vi "Logging Message Loop.vi"(8 "error in (no error)":errorcluster, 10 "Data Queue":refnum<queue>, 11 "Message Queues":T1) -> (0 "error out":errorcluster)   [LabVIEW 2019, in "Logging.lvlib"]
doc: "The message loop subVI to handle messages pertaining to logging data."
uses:
  Logging.lvlib
  support/Message Queue/All Message Queues.ctl
  support/Message Queue/Message Cluster.ctl
  controls/Components Message Queues.ctl
  Logging Configuration.ctl
  Logging State.ctl
  support/Message Queue/Enqueue Message (Single).vi
  <vilib>/Utility/error.llb/Error Cluster From Error Code.vi
  <vilib>/ErrorRing/Error Ring.xnode
  support/Message Queue/Message Queue.lvlib
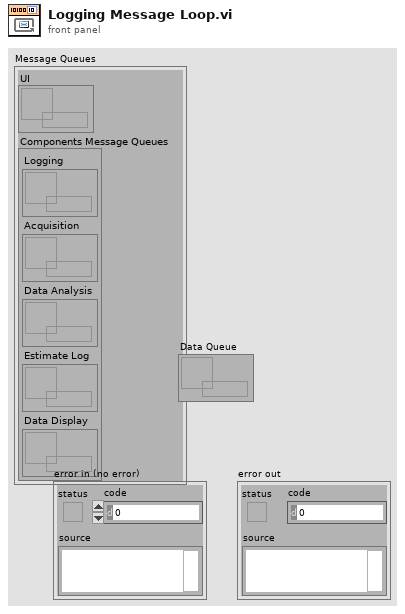
[diagram p1: front panel]
types:
  T1 = typedef "Message Queue.lvlib/All Message Queues.ctl" = cluster{"UI":refnum<queue>, "Components Message Queues":T2}
  T2 = typedef "Message Queue.lvlib/Components Message Queues.ctl" = cluster{"Logging":refnum<queue>, "Acquisition":refnum<queue>, "Data Analysis":refnum<queue>, "Estimate Log":refnum<queue>, "Data Display":refnum<queue>}
  T3 = typedef "Logging.lvlib/Logging State.ctl" = cluster{"State":enum16{"Logging", "Not Logging", "Idle"}, "Samples to Save":u32, "Force Trigger":bool}
  T4 = typedef "Logging.lvlib/Logging Configuration.ctl" = cluster{"Log File Base Path":path, "DAQ Log TDMS File Reference":refnum<k34>, "Samples to Save":u32, "Trigger - Time":u32, "Trigger - Threshold":dbl, "Trigger - Channel":u32, "Enable Time Trigger":bool, "Enable Threshold Trigger":bool, "Always Log":bool, "Session Name":string}
  T5 = enum16{"open", "open or create", "create or replace", "create", "open (read-only)"}
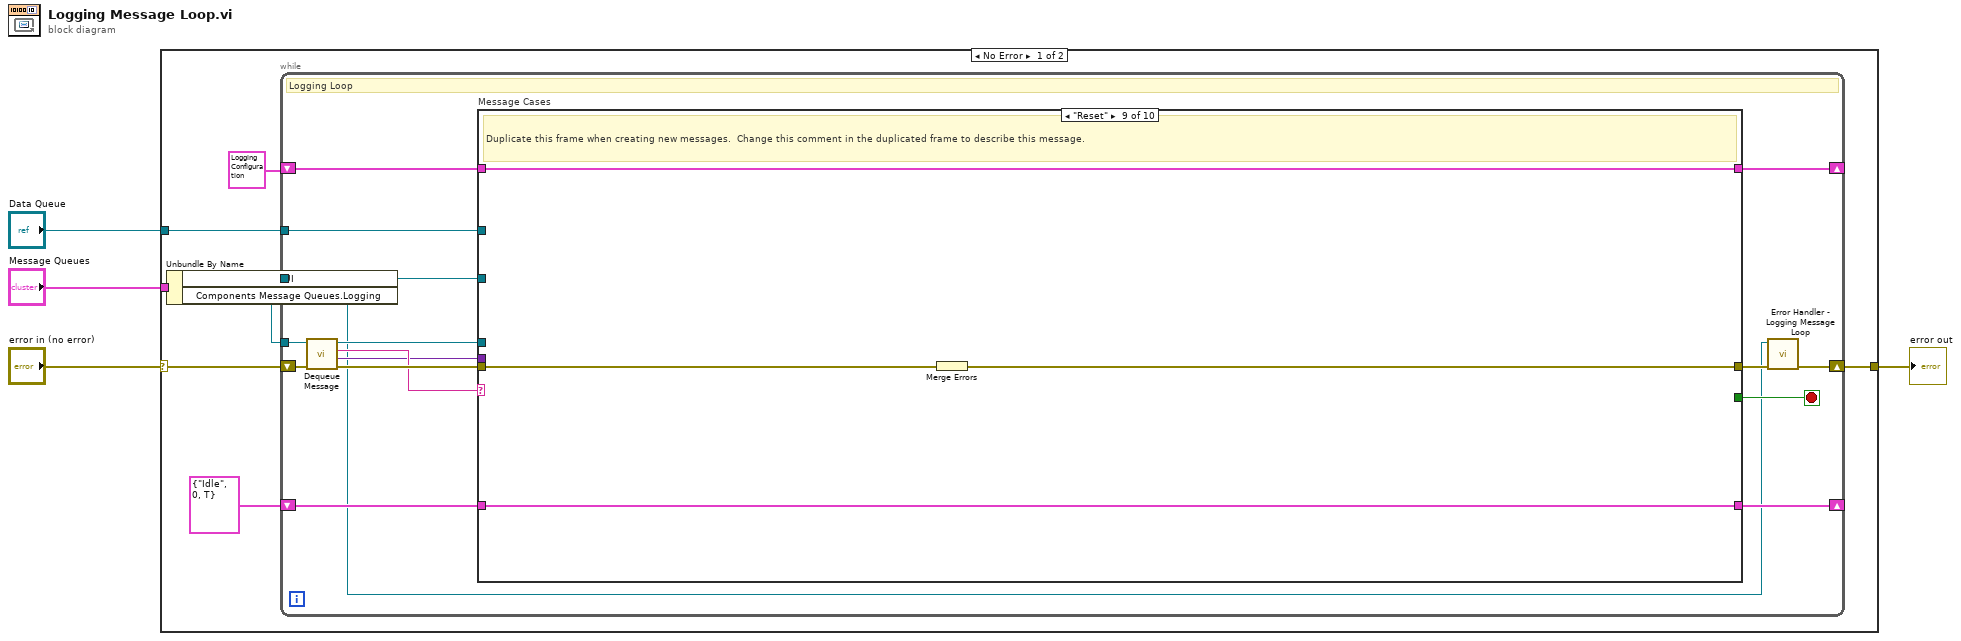
[diagram p0: block diagram]
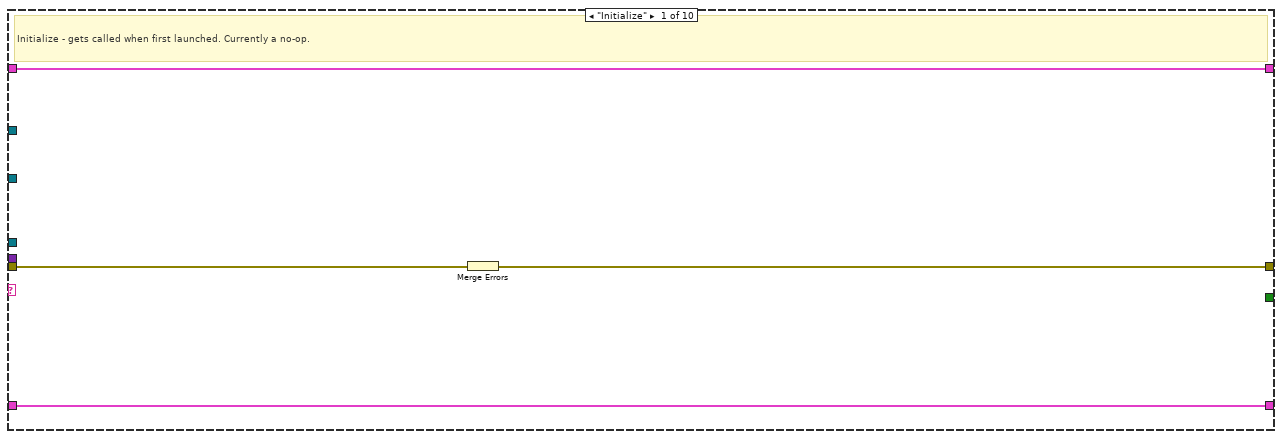
[diagram p2: hidden frame]
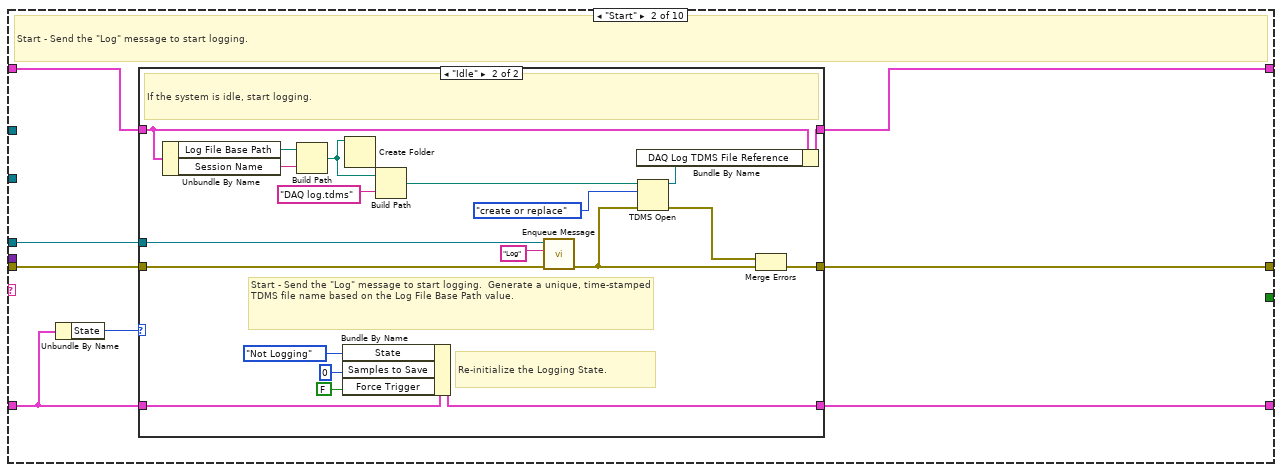
[diagram p3: hidden frame]
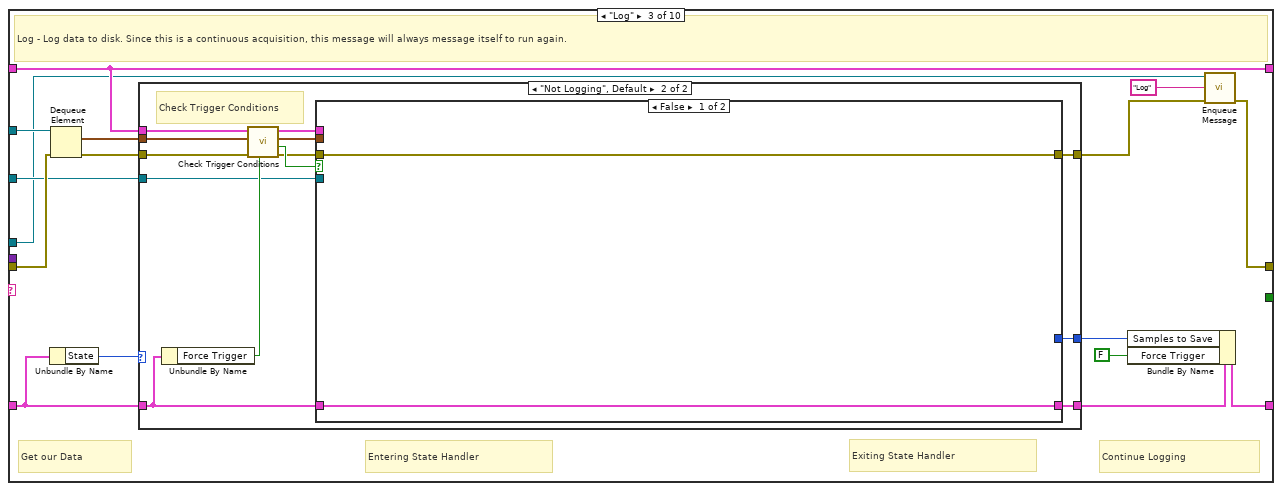
[diagram p5: hidden frame]
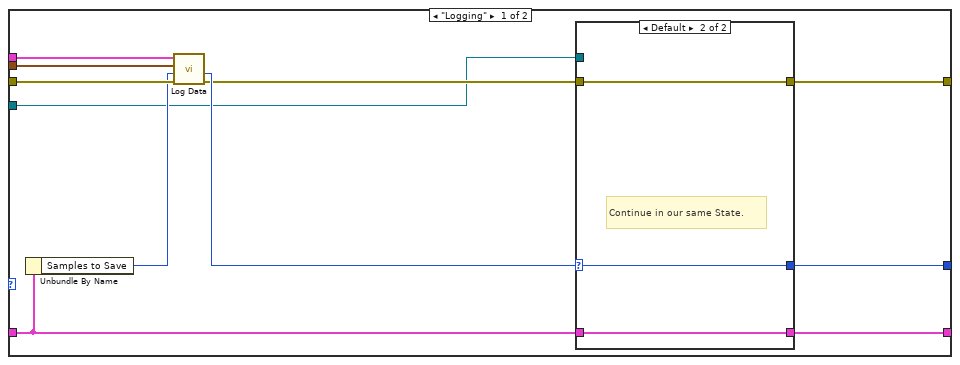
[diagram p6: hidden frame]
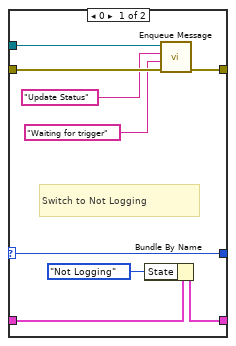
[diagram p7: hidden frame]
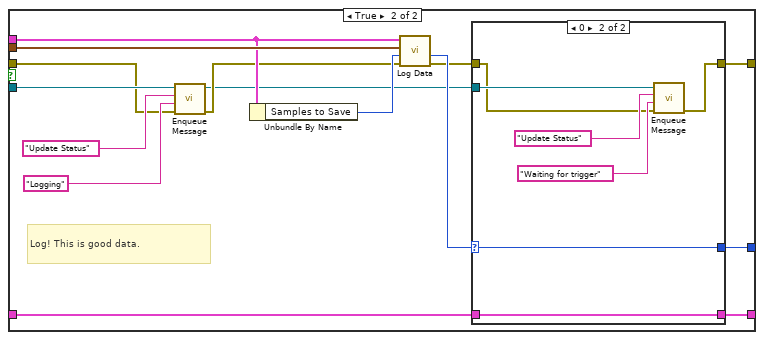
[diagram p8: hidden frame]
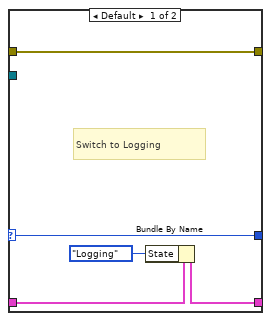
[diagram p9: hidden frame]
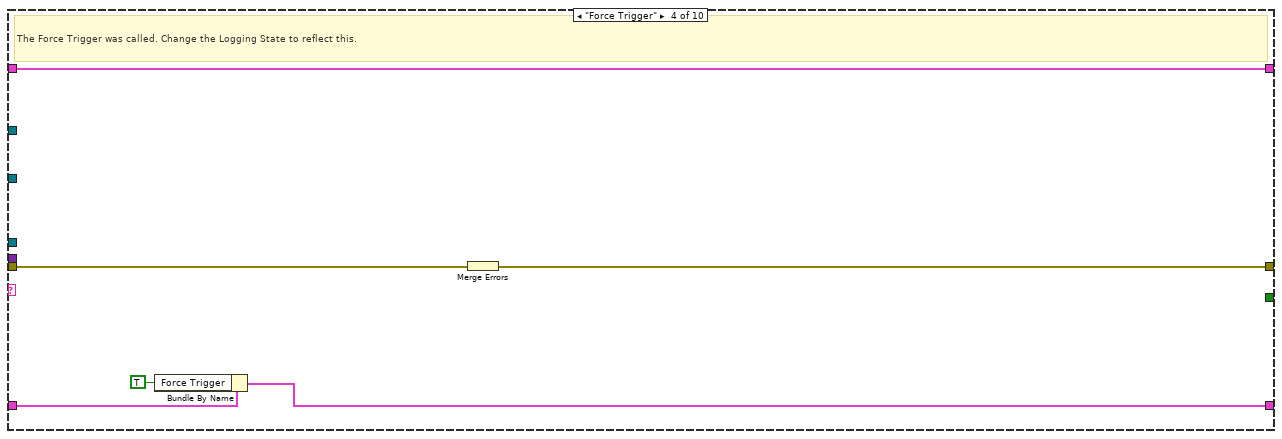
[diagram p10: hidden frame]
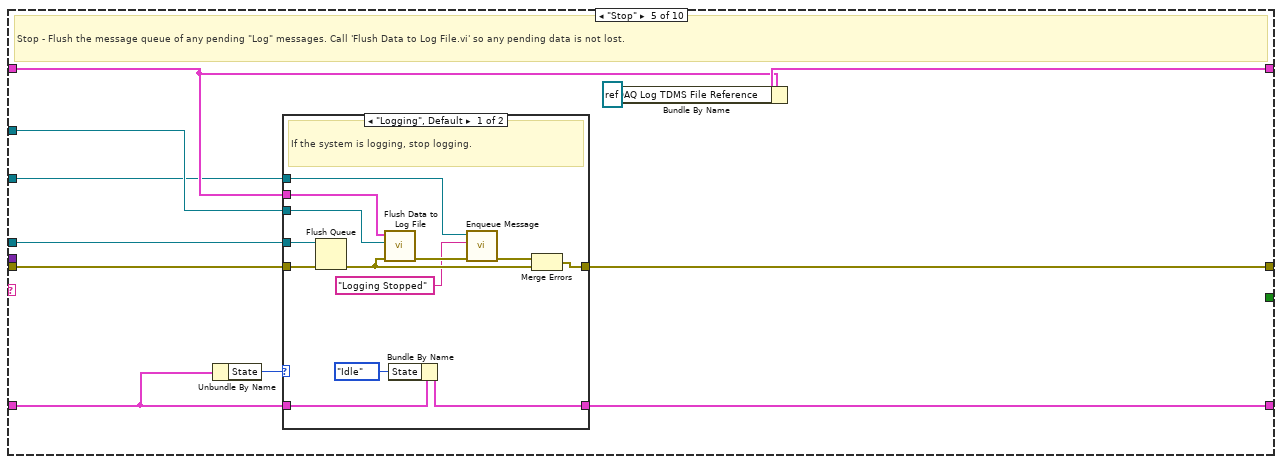
[diagram p11: hidden frame]
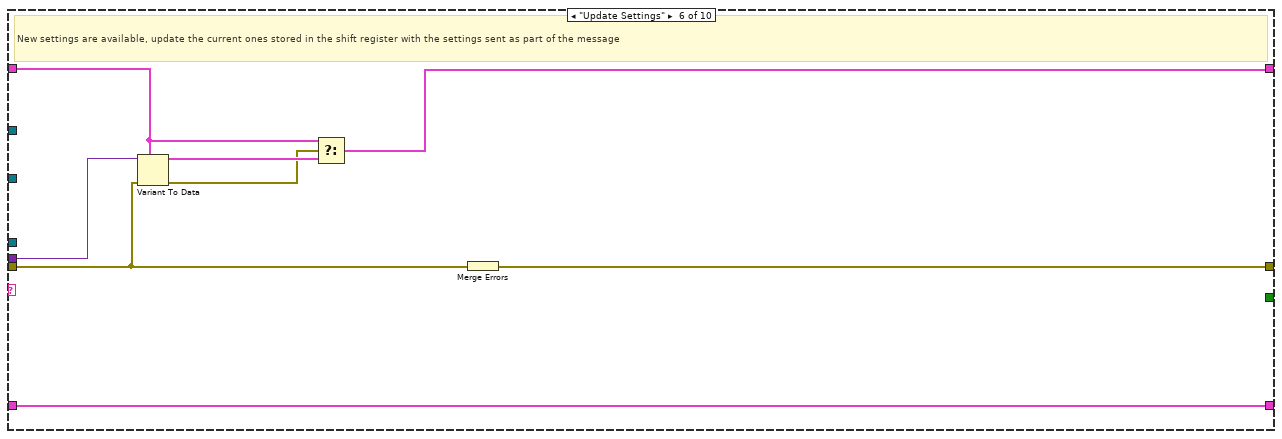
[diagram p13: hidden frame]
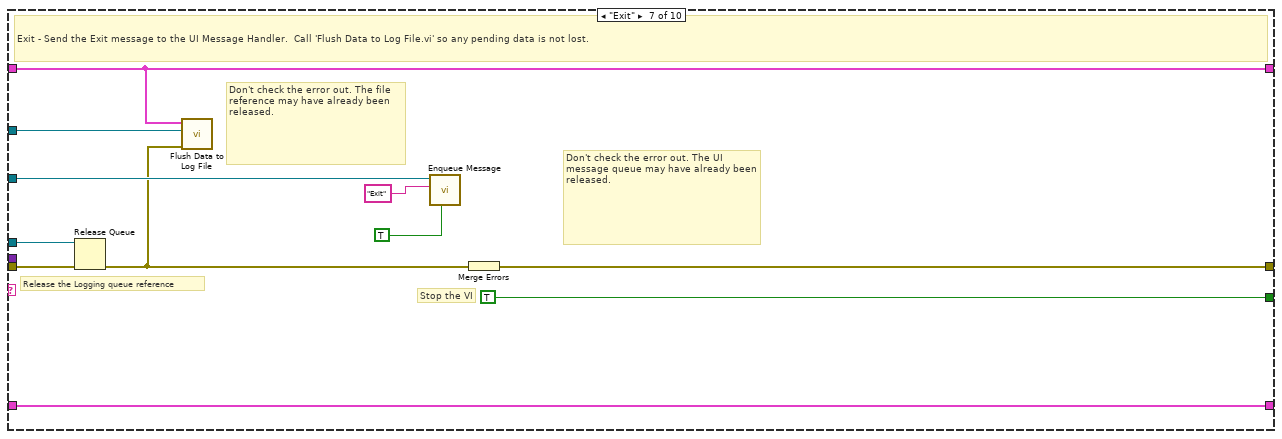
[diagram p14: hidden frame]
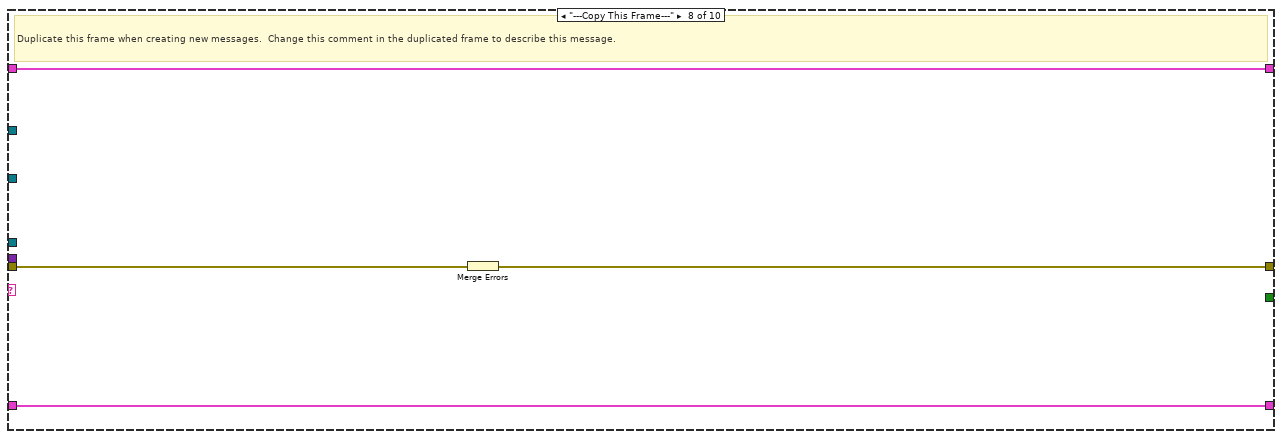
[diagram p15: hidden frame]
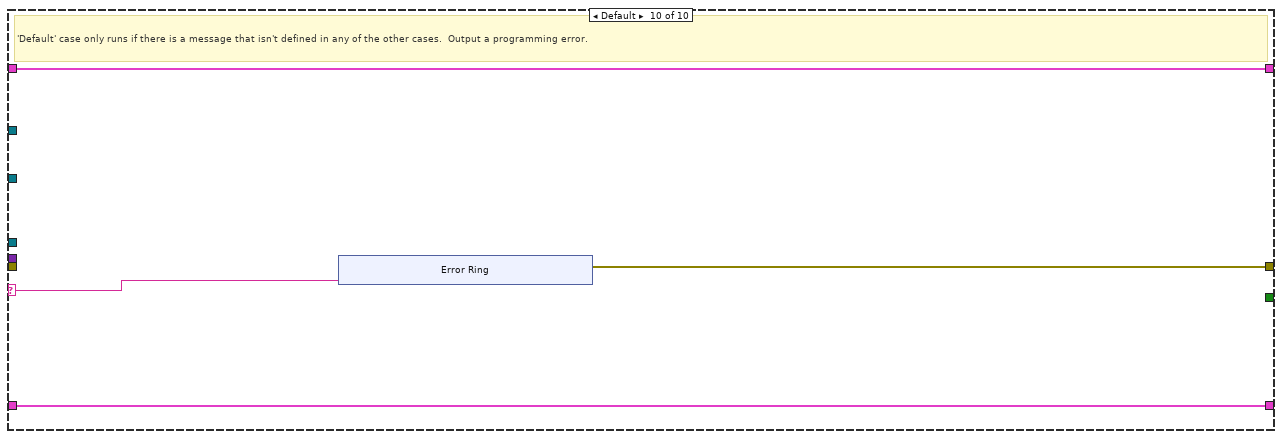
[diagram p16: hidden frame]
diagram:
  n1 = case shown="No Error" "error in (no error)" {
    selector: "error in (no error)" -> [w8 w214]
    tunnel: "Message Queues" -> [w12 _]
    tunnel: [w10 w214] -> w3
    tunnel: "Data Queue" -> [w7 _]
    frame No Error {
      n2 = Unbundle By Name(w12) -> ("UI"=w6:refnum<queue>, "Components Message Queues.Logging"=w11:refnum<queue>)
      n3 = while {
        tunnel: w11 -> [w19]
        shift-right: [w26] -> _
        shift-left: T4 {"Log File Base Path"=path "", "DAQ Log TDMS File Reference"=refnum, "Samples to Save"=0, "Trigger - Time"=0, "Trigger - Threshold"=0.0, "Trigger - Channel"=0, "Enable Time Trigger"=FALSE, "Enable Threshold Trigger"=FALSE, "Always Log"=FALSE, "Session Name"=""} ("Logging Configuration") -> [w27]
        shift-right: [w14] -> w10
        shift-left: w8 -> [w24]
        tunnel: w6 -> [w13]
        tunnel: w7 -> [w18]
        shift-right: [w16] -> _
        shift-left: T3 {"State"=enum."Idle", "Samples to Save"=0, "Force Trigger"=TRUE} -> [w17]
        stop <- w25 stop-if-true
        # "Logging Loop"
        n4 = call "Dequeue Message.vi"("error in (no error)"=w24, "Message Queue"=w19) -> ("error out"=w23:errorcluster, "Message Data"=w21:variant, "Message"=w22:string, "dup Message Queue"=w20:refnum<queue>)  [unwired: 6 in]
        n5 = case "Message Cases" shown="\"Reset\"" w22 {
          selector: w22 -> [_ _ _ _ _ _ _ _ _ w203]
          tunnel: w20 -> [_ w38 w66 _ w158 _ w188 _ _ _]
          tunnel: w23 -> [w29 w37 w76 w149 w159 w177 w191 w198 w202 _]
          tunnel: [w31 w39 w78 w147 w160 w183 w193 w196 w200 w204] -> w15
          tunnel: w27 -> [w30 w36 w71 w148 w155 w181 w187 w197 w201 w206]
          tunnel: [w30 w35 w71 w148 w157 w178 w187 w197 w201 w206] -> w26
          tunnel: [_ _ _ _ _ _ TRUE _ _ _] -> w25
          tunnel: w21 -> [_ _ _ _ _ w182 _ _ _ _]
          tunnel: w13 -> [_ _ w70 _ w153 _ w192 _ _ _]
          tunnel: w18 -> [_ _ w67 _ w154 _ w186 _ _ _]
          tunnel: w17 -> [w28 w33 w74 w146 w151 w176 w184 w195 w199 w205]
          tunnel: [w28 w34 w69 w145 w150 w176 w184 w195 w199 w205] -> w16
          frame "Initialize" {
            # "Initialize - gets called when first launched. Currently a no-op."
            n6 = Merge Errors(w29) -> (w31:errorcluster)
          }
          frame "Start" {
            # "Start - Send the \"Log\" message to start logging."
            n7 = Unbundle By Name(w33) -> ("State"=w32:enum16{"Logging", "Not Logging", "Idle"})
            n8 = case shown="\"Idle\"" w32 {
              tunnel: [w41 w62] -> w39
              tunnel: w38 -> [_ w61]
              tunnel: w37 -> [w41 w59]
              tunnel: w36 -> [w42 w58]
              tunnel: [w42 w55] -> w35
              tunnel: w33 -> [w40 w51]
              tunnel: [w40 w50] -> w34
              frame "Logging", Default {
                # "The system is already running. Ignore the \"Start\" message."
              }
              frame "Idle" {
                # "Re-initialize the Logging State."
                # "Start - Send the \"Log\" message to start logging.  Generate a unique, time-stamped TDMS file name based on the Log File Base Path value."
                # "If the system is idle, start logging."
                n9 = Unbundle By Name(w58) -> ("Log File Base Path"=w46:path, "Session Name"=w45:string)
                n10 = Build Path(base path=w46, name or relative path=w45) -> (appended path=w43:path)
                n11 = Bundle By Name(cluster=w51, "State"=enum16{"Logging", "Not Logging"}."Not Logging", "Samples to Save"=u32 0 ("Reads to Save"), "Force Trigger"=FALSE) -> (w50:T3)
                n12 = Create Folder(path (use dialog)=w43) -> ()  [unwired: 2 in, 3 out]
                n13 = Build Path(base path=w43, name or relative path="DAQ log.tdms") -> (appended path=w56:path)
                n14 = call-poly "Enqueue Message.vi"("error in (no error)"=w59, "Message"="Log", "Message Queue"=w61) -> ("error out"=w53:errorcluster)  [unwired: 7 in, 1 out]
                n15 = TDMS Open(8:w53, 10:T5."create or replace" ("operation (0:open)"), 11:w56) -> (0:w52:errorcluster, 3:w57:refnum<k34>)  [unwired: 4 in]
                n16 = Bundle By Name(cluster=w58, "DAQ Log TDMS File Reference"=w57) -> (w55:T4)
                n17 = Merge Errors(w52, w53) -> (w62:errorcluster)
              }
            }
          }
          frame "Log" {
            # "Exiting State Handler"
            # "Continue Logging"
            # "Entering State Handler"
            # "Get our Data"
            # "Log - Log data to disk. Since this is a continuous acquisition, this message will always message itself to run again."
            n18 = Unbundle By Name(w74) -> ("State"=w75:enum16{"Logging", "Not Logging", "Idle"})
            n19 = Dequeue Element(queue=w67, error in (no error)=w76) -> (element=w73:waveform(dbl)[], error out=w72:errorcluster)  [unwired: 1 in, 2 out]
            n20 = case shown="\"Not Logging\", Default" w75 {
              tunnel: [w83 w106] -> w65
              tunnel: w74 -> [w84 w104]
              tunnel: w73 -> [w88 w113]
              tunnel: w72 -> [w87 w112]
              tunnel: w71 -> [w89 w114]
              tunnel: w70 -> [w79 w103]
              tunnel: [w80 w105] -> w63
              tunnel: [w82 w102] -> w64
              frame "Logging" {
                n21 = Unbundle By Name(w84) -> ("Samples to Save"=w86:u32)
                n22 = call "Log Data.vi"("error in (no error)"=w87, "Samples to Save In"=w86, "Data"=w88, "Logging Configuration"=w89) -> ("error out"=w81:errorcluster, "Samples to Save Out"=w85:u32)  [unwired: 6 in]
                n23 = case shown="Default" w85 {
                  selector: w85 -> [w95 w101]
                  tunnel: w81 -> [w93 w100]
                  tunnel: [w94 w100] -> w80
                  tunnel: w84 -> [w97 w99]
                  tunnel: [w96 w99] -> w83
                  tunnel: [w95 w101] -> w82
                  tunnel: w79 -> [w90 _]
                  frame 0 {
                    # "Switch to Not Logging"
                    n24 = Bundle By Name(cluster=w97, "State"=enum16{"Logging", "Not Logging"}."Not Logging") -> (w96:T3)
                    n25 = call-poly "Enqueue Message.vi"("error in (no error)"=w93, "Message Data"="Waiting for trigger" ("Waiting for trigger"), "Message"="Update Status", "Message Queue"=w90) -> ("error out"=w94:errorcluster)  [unwired: 6 in, 1 out]
                  }
                  frame Default {
                    # "Continue in our same State."
                  }
                }
              }
              frame "Not Logging", Default {
                # "Check Trigger Conditions"
                n26 = Unbundle By Name(w104) -> ("Force Trigger"=w111:bool)
                n27 = call "Check Trigger Conditions.vi"("Force Trigger?"=w111, "error in (no error)"=w112, "Waveform Data In"=w113, "Logging Configuration In"=w114) -> ("error out"=w109:errorcluster, "Trigger Conditions Met?"=w110:bool, "Waveform Data Out (copy)"=w108:waveform(dbl)[], "Logging Configuration Out"=w107:T4)  [unwired: 4 in]
                n28 = case shown="False" w110 {
                  tunnel: w109 -> [w115 w125]
                  tunnel: w108 -> [_ w131]
                  tunnel: w107 -> [_ w130]
                  tunnel: w104 -> [w116 w121]
                  tunnel: [w116 w120] -> w106
                  tunnel: [w115 w118] -> w105
                  tunnel: w103 -> [_ w129]
                  tunnel: [_ w122] -> w102
                  frame False {
                  }
                  frame True {
                    # "Log! This is good data."
                    n29 = call-poly "Enqueue Message.vi"("error in (no error)"=w125, "Message Data"="Logging" ("Logging"), "Message"="Update Status", "Message Queue"=w129) -> ("error out"=w124:errorcluster, "dup Message Queue"=w117:refnum<queue>)  [unwired: 6 in]
                    n30 = Unbundle By Name(w130) -> ("Samples to Save"=w126:u32)
                    n31 = call "Log Data.vi"("error in (no error)"=w124, "Samples to Save In"=w126, "Data"=w131, "Logging Configuration"=w130) -> ("error out"=w119:errorcluster, "Samples to Save Out"=w123:u32)  [unwired: 6 in]
                    n32 = case shown="0" w123 {
                      selector: w123 -> [w136 w143]
                      tunnel: [w136 w143] -> w122
                      tunnel: [w133 w142] -> w120
                      tunnel: w121 -> [w134 w142]
                      tunnel: w119 -> [w132 w138]
                      tunnel: [w132 w137] -> w118
                      tunnel: w117 -> [_ w141]
                      frame Default {
                        # "Switch to Logging"
                        n33 = Bundle By Name(cluster=w134, "State"=enum16{"Logging", "Not Logging"}."Logging") -> (w133:T3)
                      }
                      frame 0 {
                        n34 = call-poly "Enqueue Message.vi"("error in (no error)"=w138, "Message Data"="Waiting for trigger" ("Waiting for trigger"), "Message"="Update Status", "Message Queue"=w141) -> ("error out"=w137:errorcluster)  [unwired: 6 in, 1 out]
                      }
                    }
                  }
                }
              }
            }
            n35 = Bundle By Name(cluster=w65, "Samples to Save"=w64, "Force Trigger"=FALSE) -> (w69:T3)
            n36 = call-poly "Enqueue Message.vi"("error in (no error)"=w63, "Message"="Log", "Message Queue"=w66) -> ("error out"=w78:errorcluster)  [unwired: 7 in, 1 out]
          }
          frame "Force Trigger" {
            # "The Force Trigger was called. Change the Logging State to reflect this."
            n37 = Bundle By Name(cluster=w146, "Force Trigger"=TRUE) -> (w145:T3)
            n38 = Merge Errors(w149) -> (w147:errorcluster)
          }
          frame "Stop" {
            # "Stop - Flush the message queue of any pending \"Log\" messages. Call 'Flush Data to Log File.vi' so any pending data is not lost."
            n39 = Unbundle By Name(w151) -> ("State"=w152:enum16{"Logging", "Not Logging", "Idle"})
            n40 = case shown="\"Logging\", Default" w152 {
              tunnel: [w173 w175] -> w160
              tunnel: w159 -> [w172 w175]
              tunnel: w158 -> [w171 _]
              tunnel: w155 -> [w170 _]
              tunnel: w154 -> [w169 _]
              tunnel: w153 -> [w165 _]
              tunnel: w151 -> [w163 w174]
              tunnel: [w162 w174] -> w150
              frame "Logging", Default {
                # "If the system is logging, stop logging."
                n41 = Flush Queue(queue=w171, error in (no error)=w172) -> (error out=w168:errorcluster)  [unwired: 2 out]
                n42 = call "Flush Data to Log File.vi"("error in (no error)"=w168, "Data Queue"=w169, "Logging Configuration"=w170) -> ("error out"=w167:errorcluster)  [unwired: 8 in]
                n43 = Bundle By Name(cluster=w163, "State"=enum16{"Logging", "Not Logging", "Idle"}."Idle") -> (w162:T3)
                n44 = call-poly "Enqueue Message.vi"("error in (no error)"=w167, "Message"="Logging Stopped", "Message Queue"=w165) -> ("error out"=w166:errorcluster)  [unwired: 7 in, 1 out]
                n45 = Merge Errors(w166, w168) -> (w173:errorcluster)
              }
              frame "Idle" {
                # "The system is already idle. Ignore the \"Stop\" message."
              }
            }
            n46 = Bundle By Name(cluster=w155, "DAQ Log TDMS File Reference"=refnum<k34> refnum ("tdms file out")) -> (w157:T4)
          }
          frame "Update Settings" {
            # "New settings are available, update the current ones stored in the shift register with the settings sent as part of the message"
            n47 = Variant To Data(error in=w177, type=w181, Variant=w182) -> (data=w180:T4, error out=w179:errorcluster)
            n48 = Select(t=w181, s=w179, f=w180) -> (s? t:f=w178:T4)
            n49 = Merge Errors(w177) -> (w183:errorcluster)
          }
          frame "Exit" {
            # "Don't check the error out. The file reference may have already been released."
            # "Release the Logging queue reference"
            # "Don't check the error out. The UI message queue may have already been released."
            # "Stop the VI"
            # "Exit - Send the Exit message to the UI Message Handler.  Call 'Flush Data to Log File.vi' so any pending data is not lost."
            n50 = Release Queue(queue=w188, error in (no error)=w191) -> (error out=w185:errorcluster)  [unwired: 1 in, 2 out]
            n51 = call "Flush Data to Log File.vi"("error in (no error)"=w185, "Data Queue"=w186, "Logging Configuration"=w187) -> ()  [unwired: 8 in, 1 out]
            n52 = call-poly "Enqueue Message.vi"("Priority Message? (F)"=TRUE, "Message"="Exit", "Message Queue"=w192) -> ()  [unwired: 7 in, 2 out]
            n53 = Merge Errors(w185) -> (w193:errorcluster)
          }
          frame "---Copy This Frame---" {
            # "Duplicate this frame when creating new messages.  Change this comment in the duplicated frame to describe this message."
            n54 = Merge Errors(w198) -> (w196:errorcluster)
          }
          frame "Reset" {
            # "Duplicate this frame when creating new messages.  Change this comment in the duplicated frame to describe this message."
            n55 = Merge Errors(w202) -> (w200:errorcluster)
          }
          frame Default {
            # "'Default' case only runs if there is a message that isn't defined in any of the other cases.  Output a programming error."
            n56 = xnode "Error Ring"("parameter 0"=w203) -> ("error out"=w204:errorcluster)
          }
        }
        n57 = call "Error Handler - Logging Message Loop.vi"("error in (no error)"=w15, "Message Queue"=w13) -> ("dup error in"=w14:errorcluster)  [unwired: 8 in, 1 out]
      }
    }
    frame Error {
    }
  }
  "error out" <- w3
